vi "Send Generate View Event.vi"(7 "Priority":T1=enum."Normal" caption="Message Priority (Normal)", 8 "error in (no error)":errorcluster, 10 "Event Data":refnum<class "Event.lvclass">, 11 "Message Enqueuer in":refnum<class "Message Enqueuer.lvclass">) -> (0 "error out":errorcluster, 3 "Message Enqueuer out":refnum<class "Message Enqueuer.lvclass">)   [LabVIEW 2023, in "MVC Actors.lvlib" / "Generate View Event Msg.lvclass"]
doc: "Sends the <b>MVC Actors.lvlib:Generate View Event Msg.lvclass</b> message.\n\nThis message will call <b>Generate View Event.vi</b> on the <b>MVC Actors.lvlib:View.lvclass</b> actor.\n\n<b>Generate View Event.vi Description</b>\nThis method generates/fires the Event wired to the input. Firing an event checks if the view is paused or \"Receive Only\" . This event will not be broadcast to other Views.\n\n<b>IMPORTANT</b> - Only call this method directly (i.e. without sending the corresponding message) only within the View methods. From helper loops send the corresponding message to self by calling the suitable send method. This is to make sure your View works with up-to-date settings."
uses:
  Generate View Event Msg.lvclass
  Generate View Event Msg.lvclass/Generate View Event Msg.ctl
  <vilib>/ActorFramework/Message Enqueuer/Message Enqueuer.lvclass
  C:/Program Files/National Instruments/LabVIEW 2023/vi.lib/ActorFramework/Message/Message.lvclass
  C:/Projects/Shared Libraries/Event Actors/View Messages/Generate View Event Msg/Generate View Event Msg.lvclass
  <vilib>/ActorFramework/Message Enqueuer/Message Priority.ctl
  Event/Event.lvclass
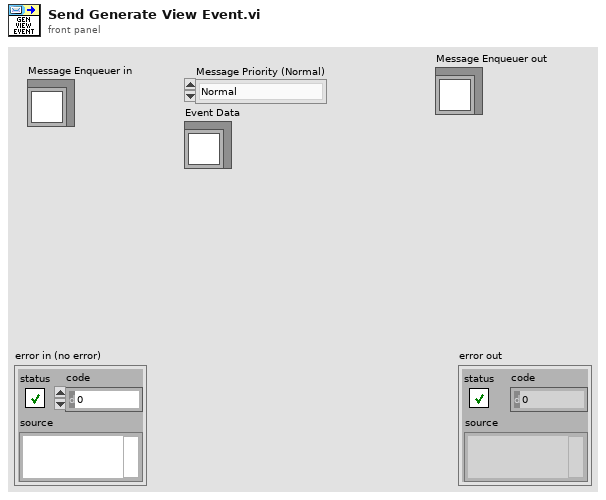
[diagram p1: front panel]
types:
  T1 = typedef "Actor Framework.lvlib/Message Enqueuer.lvclass/Message Priority.ctl" = enum16{"Low", "Normal", "High"}
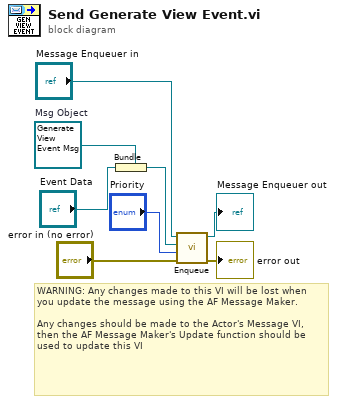
[diagram p0: block diagram]
diagram:
  w7 = refnum<class "Generate View Event Msg.lvclass"> refnum  # Msg Object
  # "WARNING: Any changes made to this VI will be lost when you update the message using the AF Message Maker.\n\nAny changes should be made to the Actor's Message VI, then the AF Message Maker's Update function should be used to update this VI"
  n1 = Bundle(cluster=w7, "Event Data") -> (w2:refnum<class "Generate View Event Msg.lvclass">)
  n2 = call <vilib>:"Enqueue.vi"("error in (no error)"="error in (no error)", "Message Priority (Normal)"="Priority", "Message"=w2, "Message Enqueuer in"="Message Enqueuer in") -> ("error out"=→"error out":errorcluster, "Message Enqueuer out"=→"Message Enqueuer out":refnum<class "Message Enqueuer.lvclass">)  [unwired: 6 in]
